vi "Processing_Logging-Loop.vi"(0 "Message Queues":T1, 5 "Unprocessed Data":refnum<queue>, 7 "Processed Data Notifier":refnum<notifier>, 9 "Control Data Notifier":refnum<notifier>, 11 "error in":errorcluster) -> (15 "error out":errorcluster)   [LabVIEW 2024]
uses:
  support/Message Queue/All Message Queues.ctl
  support/Message Queue/Message Cluster.ctl
  support/Control/Array Data Constant.ctl
  support/Control/Waveform Data Constant.ctl
  support/Control/Control Data Constant.ctl
  Logging Configuration.ctl
  Processing_Logging State.ctl
  Configuration/Calibration Configuration.ctl
  <vilib>/Utility/error.llb/Error Cluster From Error Code.vi
  <vilib>/ErrorRing/Error Ring.xnode
  support/Message Queue/Message Queue.lvlib
panel:
  out "Loop-2 Iteration Counter":i32
  out "Loop-2 Iteration Clock (ms)":u32
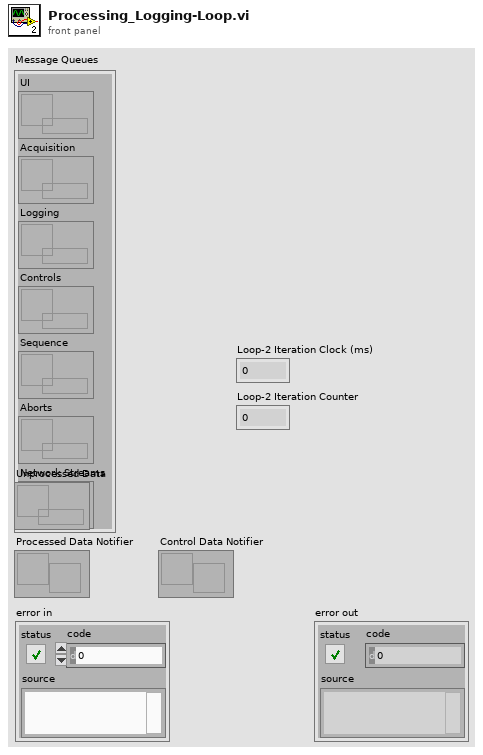
[diagram p1: front panel]
types:
  T1 = typedef "Message Queue.lvlib/All Message Queues.ctl" = cluster{"UI":refnum<queue>, "Acquisition":refnum<queue>, "Logging":refnum<queue>, "Controls":refnum<queue>, "Sequence":refnum<queue>, "Aborts":refnum<queue>, "Network Streams":refnum<queue>}
  T2 = typedef "Calibration Configuration.ctl" = cluster{"ai Calibration Slope":dbl[], "ai Calibration Offset":dbl[], "ai Sensor Names ":string[], "tc Sensor Names":string[], "di Sensor Names":string[], "do Sensor Names":string[], "bc Sensor Names":string[], "ai Sensor Units":string[], "tc Sensor Units":string[], "bc Sensor Units":string[]}
  T3 = typedef "Processing_Logging State.ctl" = enum16{"Idle", "Processing", "Logging"}
  T4 = typedef "Logging Configuration.ctl" = cluster{"Data File Name":string, "TDMS File Reference":refnum<k34>}
  T5 = typedef "Data Constant.ctl" = cluster{"AI":dbl[][], "AIraw":dbl[][], "TC":dbl[][], "BC":dbl[][], "DI":dbl[][], "DI2":dbl[][], "DO":dbl[][], "t (local)":dbl}
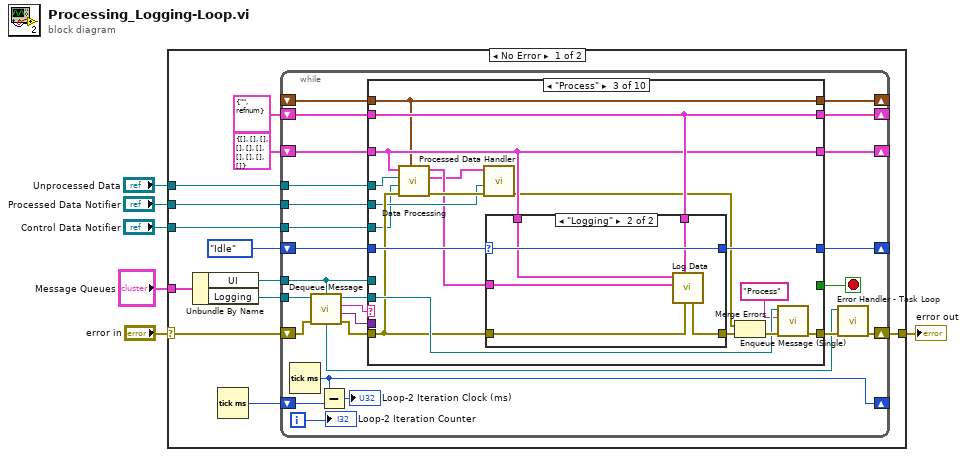
[diagram p0: block diagram]
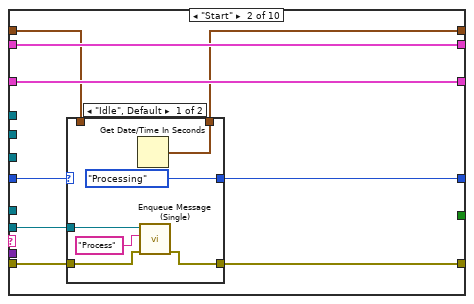
[diagram p3: hidden frame]
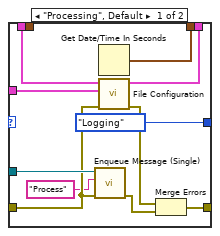
[diagram p7: hidden frame]
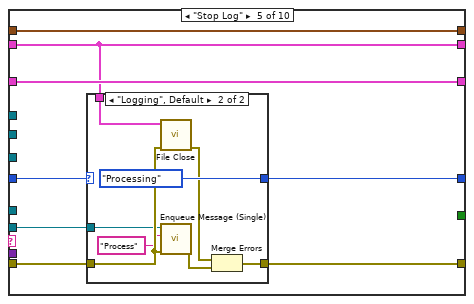
[diagram p8: hidden frame]
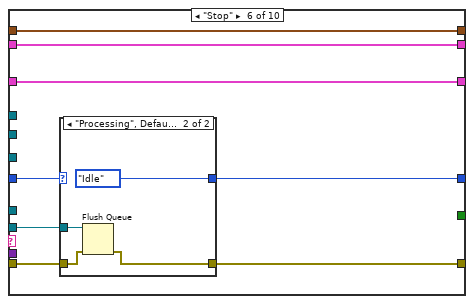
[diagram p10: hidden frame]
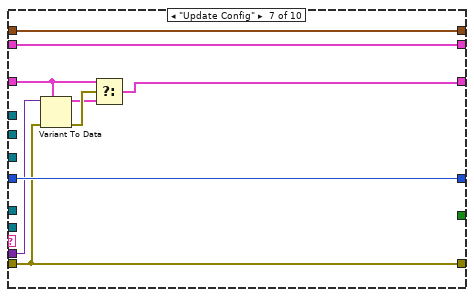
[diagram p12: hidden frame]
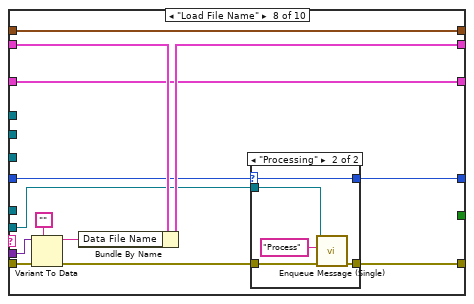
[diagram p13: hidden frame]
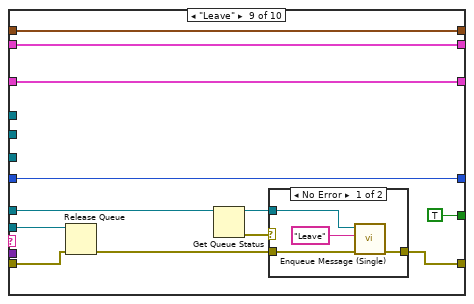
[diagram p15: hidden frame]
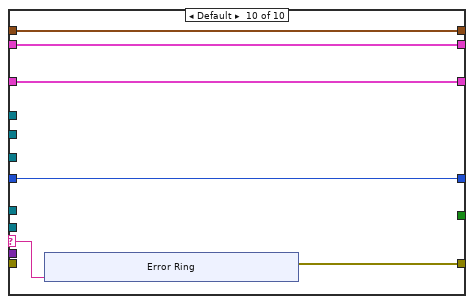
[diagram p17: hidden frame]
diagram:
  n1 = case shown="No Error" "error in" {
    selector: "error in" -> [w18 w209]
    tunnel: [w17 w209] -> w5
    tunnel: "Message Queues" -> [w13 _]
    tunnel: "Unprocessed Data" -> [w15 _]
    tunnel: "Processed Data Notifier" -> [w14 _]
    tunnel: "Control Data Notifier" -> [w7 _]
    frame No Error {
      n2 = Unbundle By Name(w13) -> ("UI"=w12:refnum<queue>, "Logging"=w11:refnum<queue>)
      n3 = Tick Count (ms)() -> (millisecond timer value=w9:u32)
      n4 = while {
        shift-right: [w43] -> w17
        shift-left: w18 -> [w41]
        shift-right: [w33] -> _
        shift-left: T2 {"ai Calibration Slope"=[], "ai Calibration Offset"=[], "ai Sensor Names "=[], "tc Sensor Names"=[], "di Sensor Names"=[], "do Sensor Names"=[], "bc Sensor Names"=[], "ai Sensor Units"=[], "tc Sensor Units"=[], "bc Sensor Units"=[]} ("Calibration Configuration") -> [w22]
        shift-right: [w32] -> _
        shift-left: T4 {"Data File Name"="", "TDMS File Reference"=refnum} ("Logging Configuration") -> [w34]
        tunnel: w15 -> [w28]
        tunnel: w14 -> [w27]
        tunnel: w12 -> [w35]
        tunnel: w11 -> [w42]
        shift-right: [w30] -> _
        shift-left: Processing_Logging_State."Idle" ("Porcess/Log State") -> [w31]
        shift-right: [w24] -> _
        shift-left: w9 -> [w25]
        shift-right: [w21] -> _
        shift-left: _ -> [w20]
        tunnel: w7 -> [w19]
        i -> [w23]
        stop <- w29 stop-if-true
        n5 = Tick Count (ms)() -> (millisecond timer value=w24:u32)
        n6 = call "Dequeue Message.vi"("error in (no error)"=w41, "Message Queue"=w42) -> ("error out"=w40:errorcluster, "Message Data"=w36:variant, "Message"=w37:string, "dup Message Queue"=w38:refnum<queue>)  [unwired: 6 in]
        n7 = Subtract(x=w24, y=w25) -> (x-y=→"Loop-2 Iteration Clock (ms)":u32)
        n8 = case shown="\"Process\"" w37 {
          selector: w37 -> [_ _ _ _ _ _ _ _ _ w198]
          tunnel: w35 -> [_ _ _ _ _ _ _ _ w184 _]
          tunnel: w40 -> [w45 w54 w76 w100 w121 w139 w156 w171 w186 _]
          tunnel: [w45 w53 w79 w99 w120 w138 w156 w161 w183 w199] -> w39
          tunnel: w38 -> [_ w52 w78 w98 w124 w140 _ w163 w187 _]
          tunnel: w36 -> [_ _ _ _ _ _ w155 w170 _ _]
          tunnel: w34 -> [w47 w51 w82 w96 w119 w137 w153 w168 w189 w200]
          tunnel: w22 -> [w48 w57 w75 w93 w125 w143 w152 w165 w190 w201]
          tunnel: [w48 w57 w75 w93 w125 w143 w158 w165 w190 w201] -> w33
          tunnel: [w47 w51 w82 w97 w119 w137 w153 w167 w189 w200] -> w32
          tunnel: w31 -> [w46 w56 w84 w102 w122 w142 w157 w164 w188 w197]
          tunnel: [w46 w55 w83 w101 w123 w141 w157 w160 w188 w197] -> w30
          tunnel: [_ _ _ _ _ _ _ _ TRUE _] -> w29
          tunnel: w28 -> [_ _ w67 _ _ _ _ _ _ _]
          tunnel: w27 -> [_ _ w72 _ _ _ _ _ _ _]
          tunnel: [w44 w50 w69 w94 w118 w136 w150 w159 w182 w196] -> w21
          tunnel: w20 -> [w44 w49 w69 w95 w118 w136 w150 w159 w182 w196]
          tunnel: w19 -> [_ _ w68 _ _ _ _ _ _ _]
          frame "Initialize" {
          }
          frame "Start" {
            n9 = case shown="\"Idle\", Default" w56 {
              selector: w56 -> [_ w66]
              tunnel: [Processing_Logging_State."Processing" ("Porcess/Log State") w66] -> w55
              tunnel: w54 -> [w63 w65]
              tunnel: [w59 w65] -> w53
              tunnel: w52 -> [w61 _]
              tunnel: [w58 w64] -> w50
              tunnel: w49 -> [_ w64]
              frame "Idle", Default {
                n10 = Get Date/Time In Seconds() -> (seconds since 1Jan1904=w58:timestamp)
                n11 = call "Enqueue Message (Single).vi"("error in (no error)"=w63, "Message"="Process", "Message Queue"=w61) -> ("error out"=w59:errorcluster)  [unwired: 7 in, 1 out]
              }
              frame "Processing" {
              }
            }
          }
          frame "Process" {
            n12 = call "Data Processing.vi"("Start Time Stamp"=w69, "error in"=w76, "Control Data Notifier"=w68, "Unprocessed Data"=w67, "Calibration Configuration"=w75) -> ("error out"=w73:errorcluster, "Data"=w70:T5, "Data w Time"=w71:T5)  [unwired: 4 in]
            n13 = call "Processed Data Handler.vi"("error in"=w73, "Processed Data Notifier"=w72, "Data"=w70) -> ("error out"=w74:errorcluster)  [unwired: 8 in]
            n14 = case shown="\"Logging\"" w84 {
              selector: w84 -> [w86 w92]
              tunnel: [w86 w92] -> w83
              tunnel: w82 -> [_ w91]
              tunnel: w76 -> [w85 w90]
              tunnel: [w85 w89] -> w81
              tunnel: w75 -> [_ w88]
              tunnel: w71 -> [_ w87]
              frame "Processing", Default {
              }
              frame "Logging" {
                n15 = call "Log Data.vi"("error in (no error)"=w90, "Logging Configuration"=w91, "Data w Time"=w87, "Calibration Configuration"=w88) -> ("error out"=w89:errorcluster)  [unwired: 7 in]
              }
            }
            n16 = Merge Errors(w74, w81) -> (w80:errorcluster)
            n17 = call "Enqueue Message (Single).vi"("error in (no error)"=w80, "Message"="Process", "Message Queue"=w78) -> ("error out"=w79:errorcluster)  [unwired: 7 in, 1 out]
          }
          frame "Start Log" {
            n18 = case shown="\"Logging\"" w102 {
              selector: w102 -> [_ w117]
              tunnel: [Processing_Logging_State."Logging" ("Porcess/Log State") w117] -> w101
              tunnel: w100 -> [w111 w116]
              tunnel: [w109 w116] -> w99
              tunnel: w98 -> [w112 _]
              tunnel: w96 -> [w106 w115]
              tunnel: [w105 w115] -> w97
              tunnel: w95 -> [_ w114]
              tunnel: [w104 w114] -> w94
              tunnel: w93 -> [w103 _]
              frame "Processing", Default {
                n19 = call "Enqueue Message (Single).vi"("error in (no error)"=w111, "Message"="Process", "Message Queue"=w112) -> ("error out"=w108:errorcluster)  [unwired: 7 in, 1 out]
                n20 = Get Date/Time In Seconds() -> (seconds since 1Jan1904=w104:timestamp)
                n21 = call "File Configuration.vi"("error in"=w111, "Calibration Configuration"=w103, "Logging Configuration in"=w106) -> ("error out"=w107:errorcluster, "Logging Configuration out"=w105:T4)  [unwired: 7 in]
                n22 = Merge Errors(w107, w108) -> (w109:errorcluster)
              }
              frame "Logging" {
              }
            }
          }
          frame "Stop Log" {
            n23 = case shown="\"Logging\", Default" w122 {
              selector: w122 -> [w127 _]
              tunnel: [w127 Processing_Logging_State."Processing" ("Porcess/Log State")] -> w123
              tunnel: w121 -> [w126 w135]
              tunnel: [w126 w130] -> w120
              tunnel: w124 -> [_ w133]
              tunnel: w119 -> [_ w131]
              frame "Processing" {
              }
              frame "Logging", Default {
                n24 = call "File Close.vi"("error in (no error)"=w135, "Logging Configuration"=w131) -> ("error out"=w129:errorcluster)  [unwired: 9 in]
                n25 = call "Enqueue Message (Single).vi"("error in (no error)"=w135, "Message"="Process", "Message Queue"=w133) -> ("error out"=w128:errorcluster)  [unwired: 7 in, 1 out]
                n26 = Merge Errors(w129, w128) -> (w130:errorcluster)
              }
            }
          }
          frame "Stop" {
            n27 = case shown="\"Processing\", Default" w142 {
              selector: w142 -> [w145 _]
              tunnel: [w145 Processing_Logging_State."Idle" ("Porcess/Log State")] -> w141
              tunnel: w140 -> [_ w148]
              tunnel: w139 -> [w144 w147]
              tunnel: [w144 w146] -> w138
              frame "Idle" {
              }
              frame "Processing", Default {
                n28 = Flush Queue(queue=w148, error in (no error)=w147) -> (error out=w146:errorcluster)  [unwired: 2 out]
              }
            }
          }
          frame "Update Config" {
            n29 = Variant To Data(error in=w156, type=w152, Variant=w155) -> (data=w151:T2, error out=w154:errorcluster)
            n30 = Select(t=w152, s=w154, f=w151) -> (s? t:f=w158:T2)
          }
          frame "Load File Name" {
            n31 = Variant To Data(error in=w171, type="", Variant=w170) -> (data=w166:string, error out=w162:errorcluster)
            n32 = Bundle By Name(cluster=w168, "Data File Name"=w166) -> (w167:T4)
            n33 = case shown="\"Processing\"" w164 {
              selector: w164 -> [w173 w175]
              tunnel: w163 -> [_ w178]
              tunnel: w162 -> [w172 w177]
              tunnel: [w172 w176] -> w161
              tunnel: [w173 w175] -> w160
              frame "Idle", Default {
              }
              frame "Processing" {
                n34 = call "Enqueue Message (Single).vi"("error in (no error)"=w177, "Message"="Process", "Message Queue"=w178) -> ("error out"=w176:errorcluster)  [unwired: 7 in, 1 out]
              }
            }
          }
          frame "Leave" {
            n35 = Release Queue(queue=w187, error in (no error)=w186) -> (error out=w180:errorcluster)  [unwired: 1 in, 2 out]
            n36 = Get Queue Status(queue=w184) -> (queue out=w181:refnum<queue>, error out=w179:errorcluster)  [unwired: 2 in, 6 out]
            n37 = case shown="No Error" w179 {
              tunnel: [w193 w195] -> w183
              tunnel: w181 -> [w192 _]
              tunnel: w180 -> [w191 w195]
              frame No Error {
                n38 = call "Enqueue Message (Single).vi"("error in (no error)"=w191, "Message"="Leave", "Message Queue"=w192) -> ("error out"=w193:errorcluster)  [unwired: 7 in, 1 out]
              }
              frame Error {
              }
            }
          }
          frame Default {
            n39 = xnode "Error Ring"("parameter 0"=w198) -> ("error out"=w199:errorcluster)
          }
        }
        n40 = call "Error Handler - Task Loop.vi"("error in (no error)"=w39, "Message Queue"=w35) -> ("dup error in"=w43:errorcluster)  [unwired: 8 in, 1 out]
        "Loop-2 Iteration Counter" <- w23
      }
    }
    frame Error {
    }
  }
  "error out" <- w5
